vi "ConvertStrings(Normal to Hex).vi"(11 "Byte array":string[](array[string])) -> (3 "Hexadecimal command string":string)   [LabVIEW 2010]
panel:
  out "Decimal value":u8
  out "ASCII Output":string
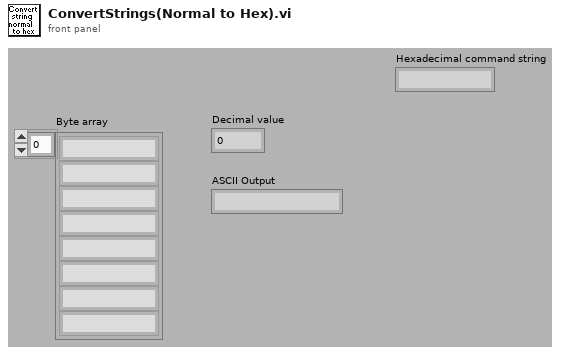
[diagram p1: front panel]
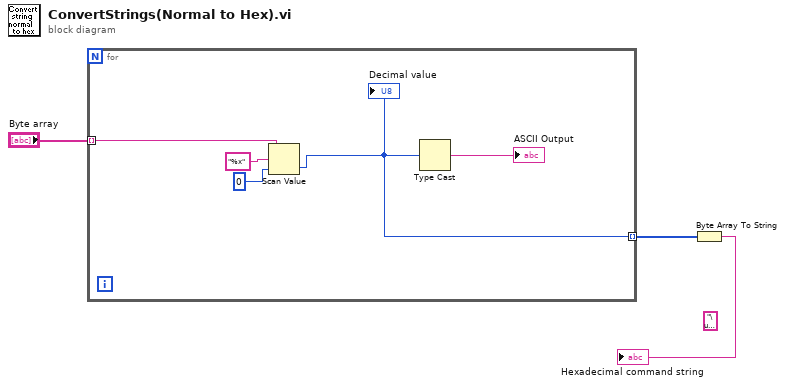
[diagram p0: block diagram]
diagram:
  (unwired) "\u000f" ("Hexadecimal command string")
  n1 = for {
    tunnel: [w5] -> w3 mode=indexing
    tunnel: "Byte array" -> [w4] mode=indexing
    n2 = Scan Value(string=w4, format string="%x", default (0 dbl)=u8 0 ("number")) -> (value=w5:u8)  [unwired: 1 out]
    "Decimal value" <- w5
    n3 = Type Cast(x=w5) -> (*(type *) &x=→"ASCII Output":string)  [unwired: 1 out]
  }
  n4 = Byte Array To String(unsigned byte array=w3) -> (string=→"Hexadecimal command string":string)
